vi "Write Binary Data.vi"(8 "error in (no error)":errorcluster, 9 "Binary Data":u8[](array[numeric]), 10 "Device Data Model":refnum<class "WebSocket Data Model.lvclass">, 11 "WebSocket in":refnum<class "WebSocket.lvclass">) -> (0 "error out":errorcluster, 3 "WebSocket out":refnum<class "WebSocket.lvclass">)   [LabVIEW 2021, in "WebSockets.lvlib" / "WebSocket.lvclass"]
doc: "Writes a binary frame to the WebSocket connection endpoint.\nWebSockets 2.0.1.40\nSam Sharp - MediaMongrels Ltd\nCopyright (c) 2019, MediaMongrels Ltd"
uses:
  WebSocket.lvclass
  Data Model/WebSocket Data Model.lvclass
  Opcodes.ctl
  WebSocket.lvclass/WebSocket.ctl
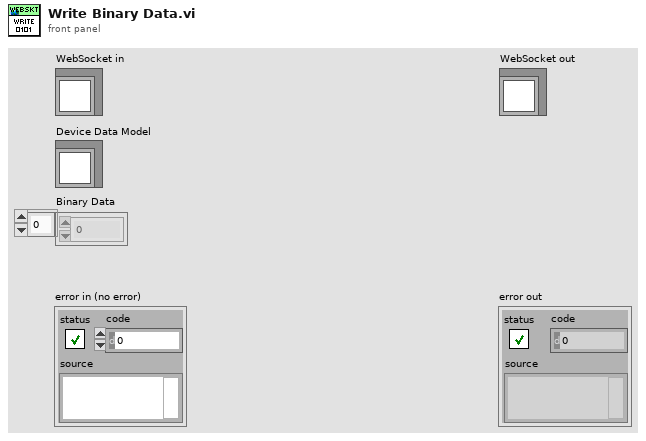
[diagram p1: front panel]
types:
  T1 = typedef "WebSockets.lvlib/WebSocket.lvclass/Opcodes.ctl" = u8
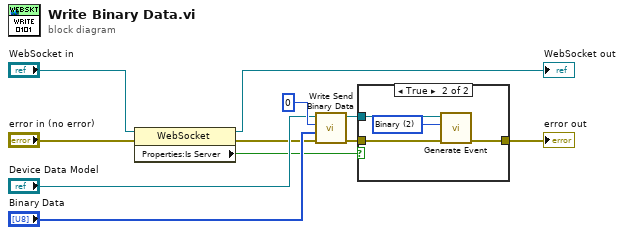
[diagram p0: block diagram]
diagram:
  n1 = property class="WebSocket"(reference="WebSocket in", error in="error in (no error)") -> (reference out=→"WebSocket out":refnum<class "WebSocket.lvclass">, error out=w4:errorcluster, "Properties:Is Server"=w1:bool)
  n2 = call-dynamic "Write Send Binary Data.vi"("error in (no error)"=w4, "values"="Binary Data", "starting address"=u16 0, "standard data model in"="Device Data Model") -> ("error out"=w6:errorcluster, "standard data model out"=w7:refnum<class "WebSocket Data Model.lvclass">)  [unwired: 6 in]
  n3 = case shown="True" w1 {
    tunnel: w7 -> [_ w15]
    tunnel: w6 -> [w12 w16]
    tunnel: [w12 w13] -> w2
    frame False {
    }
    frame True {
      w14 = T1 2 items=["Cont. Frame"=0, "Text"=1, "Binary"=2, "Close Frame"=8, "Ping"=9, "Pong"=10] ("opcode (text)")
      n4 = call "Generate Event.vi"("error in (no error)"=w16, "opcode (text)"=w14, "device data model in"=w15) -> ("error out"=w13:errorcluster)  [unwired: 7 in, 1 out]
    }
  }
  "error out" <- w2
